vi "Read Data Bit Error Rate.vi"(8 "error in (no error)":errorcluster, 10 "Bit Error Rate Options (0: Bit Error Count)":i32(ring) items=["Bit Error Count", "Bit Count", "Bit Error Rate", "All", "Total Bit Error Count", "Total Bit Count", "Total Bit Error Rate", "Judge"], 11 "VISA resource name":refnum<visa-resource-name>) -> (0 "error out":errorcluster, 1 "Judge Pass Fail Result":string, 2 "Data Measurement":dbl, 3 "VISA resource name out":refnum<visa-resource-name>)   [LabVIEW 2018, in "Agilent PSG MXG Series.lvlib"]
doc: "Fetches the data measurement for the selected measurements of bit error rate.\n\n<b>Note:</b>\nIt is applicable for N5172B/82B with <b>Option UN7</b> only."
uses:
  Agilent PSG MXG Series.lvlib
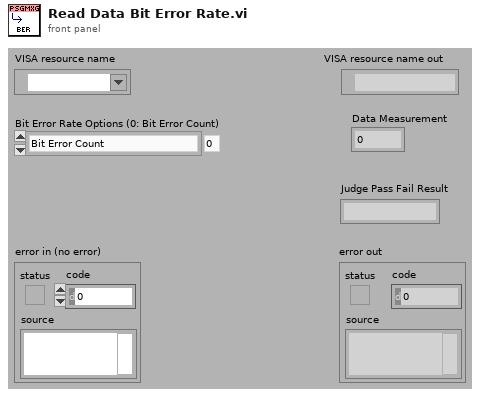
[diagram p1: front panel]
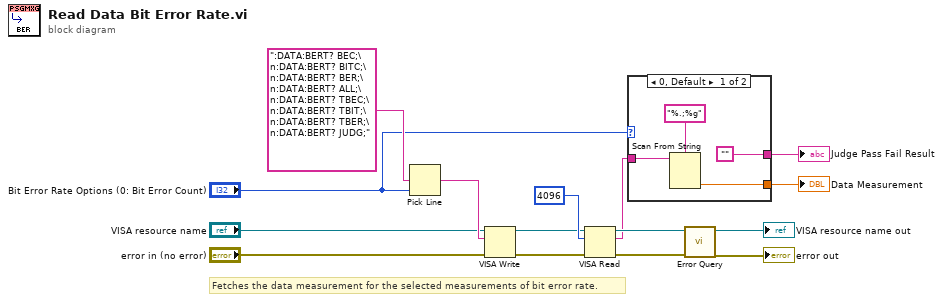
[diagram p0: block diagram]
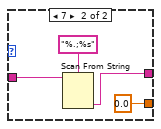
[diagram p2: hidden frame]
diagram:
  # "Fetches the data measurement for the selected measurements of bit error rate."
  n1 = Pick Line(multi-line string=":DATA:BERT? BEC;\n:DATA:BERT? BITC;\n:DATA:BERT? BER;\n:DATA:BERT? ALL;\n:DATA:BERT? TBEC;\n:DATA:BERT? TBIT;\n:DATA:BERT? TBER;\n:DATA:BERT? JUDG;", line index="Bit Error Rate Options (0: Bit Error Count)") -> (output string=w14:string)  [unwired: 1 in]
  n2 = VISA Write(VISA resource name="VISA resource name", write buffer=w14, error in (no error)="error in (no error)") -> (VISA resource name out=w10:refnum<visa-resource-name>, error out=w9:errorcluster)  [unwired: 1 out]
  n3 = VISA Read(VISA resource name=w10, byte count=u32 4096, error in (no error)=w9) -> (VISA resource name out=w8:refnum<visa-resource-name>, read buffer=w4:string, error out=w7:errorcluster)  [unwired: 1 out]
  n4 = case shown="0, Default" "Bit Error Rate Options (0: Bit Error Count)" {
    tunnel: w4 -> [w18 w22]
    tunnel: [w17 0.0] -> w2
    tunnel: ["" w21] -> w1
    frame 0, Default {
      n5 = Scan From String(format string="%.;%g", input string=w18) -> (output 1=w17:dbl)  [unwired: 3 in, 3 out]
    }
    frame 7 {
      n6 = Scan From String(format string="%.;%s", input string=w22) -> (output 1=w21:string)  [unwired: 3 in, 3 out]
    }
  }
  "Data Measurement" <- w2
  "Judge Pass Fail Result" <- w1
  n7 = call "Error Query.vi"("error in (no error)"=w7, "VISA resource name"=w8) -> ("error out"=→"error out":errorcluster, "VISA resource name out"=→"VISA resource name out":refnum<visa-resource-name>)  [unwired: 6 in, 2 out]
